vi "Digital Audio Protocol Settings Dialog.vi"() -> (3 "digital audio protocol settings":T1={"number of channels"=0, "data justification"=enum."Left Justified", "endianness"=enum."LSB First", "channel length"=0, "bit depth"=0, "frame clock rate"=0.0, "bit clock edge sync"=enum."Falling", "master clock rate"=0.0, "Logic Level"=enum."1.2 V", "frame sync edge for channel 0"=enum."Rising", "Channel 0 Offset"=0})   [LabVIEW 2021]
uses:
  digital audio protocol settings.ctl
  <vilib>/PDM Acquisition Toolkit/shared/controls/PCM Data Justification.ctl
  <vilib>/PDM Acquisition Toolkit/shared/controls/PCM Bit Endianness.ctl
  <vilib>/PDM Acquisition Toolkit/shared/controls/Digital Edge.ctl
  <vilib>/PDM Acquisition Toolkit/host/Classes/Session/Controls/Logic Levels.ctl
  Program Files/National Instruments/LabVIEW 2021/examples/Digital Audio Acquisition and Generation Toolkit/subVIs/PCM Interface Type.ctl
  <vilib>/PDM Acquisition Toolkit/shared/PDM Shared.lvlib
  <vilib>/PDM Acquisition Toolkit/host/Classes/Session/DecoderSession.lvclass
panel:
  in  "Logic level":enum8{"3.3 V", "1.8 V", "1.2 V"}(ring)=enum."1.8 V"
  in  "Master clock rate":dbl=64.0 format="%#_6pHz"
  out "Bit clock rate":dbl=64.0 format="%#_6pHz"
  in  "Number of channels":u8=2
  in  "TDM":bool
  in  "RJ":bool
  in  "LJ":bool
  in  "I2S":bool
  in  "Bit clock edge  sync":enum8{"Rising", "Falling"}(ring)=enum."Falling"
  in  "Frame clock rate":dbl=64.0 format="%#_6pHz"
  in  "Data Justification":enum16{"Left Justified", "Right Justified"}(ring) caption="Data justification"
  in  "Endianness":enum16{"MSB First", "LSB First"}(ring)
  in  "Bit depth":u8=24
  in  "Channel length":u16=32
  in  "Frame sync edge for Channel 0":enum16{"Rising", "Falling"}(ring)=enum."Falling"
  # "Protocols"
  # "Audio Configuration"
  # "Clock Configuration"
  # "Signal Configuration"
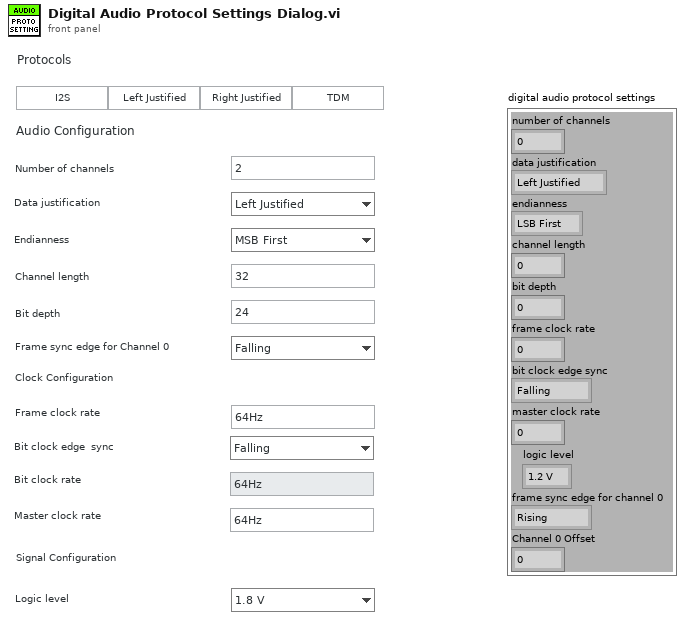
[diagram p1: front panel]
types:
  T1 = typedef "digital audio protocol settings.ctl" = cluster{"number of channels":u16, "data justification":T2, "endianness":T3, "channel length":u16, "bit depth":u8, "frame clock rate":dbl, "bit clock edge sync":T4, "master clock rate":dbl, "Logic Level":T5, "frame sync edge for channel 0":T4, "Channel 0 Offset":u16}
  T2 = typedef "PDM Shared.lvlib/PCM Data Justification.ctl" = enum16{"Left Justified", "Right Justified"}
  T3 = typedef "PDM Shared.lvlib/PCM Bit Endianness.ctl" = enum16{"MSB First", "LSB First"}
  T4 = typedef "PDM Shared.lvlib/Digital Edge.ctl" = enum8{"Rising", "Falling"}
  T5 = typedef "PDM Acquisition Class Library.lvlib/DecoderSession.lvclass/Logic Levels.ctl" = enum16{"3.3 V", "1.8 V", "1.2 V"}
  T6 = enum32{"Invalid", "Standard", "Closed", "Hidden", "Minimized", "Maximized"}
  T7 = typedef "PCM Interface Type.ctl" = enum16{"I2S", "Left Justified", "Right Justified", "TDM 4 Channel", "TDM 6 Channel", "TDM 8 Channel", "DSP mode", "DSP mode with 1 bit delay", "PCM Short Frame", "PCM Long Frame"}
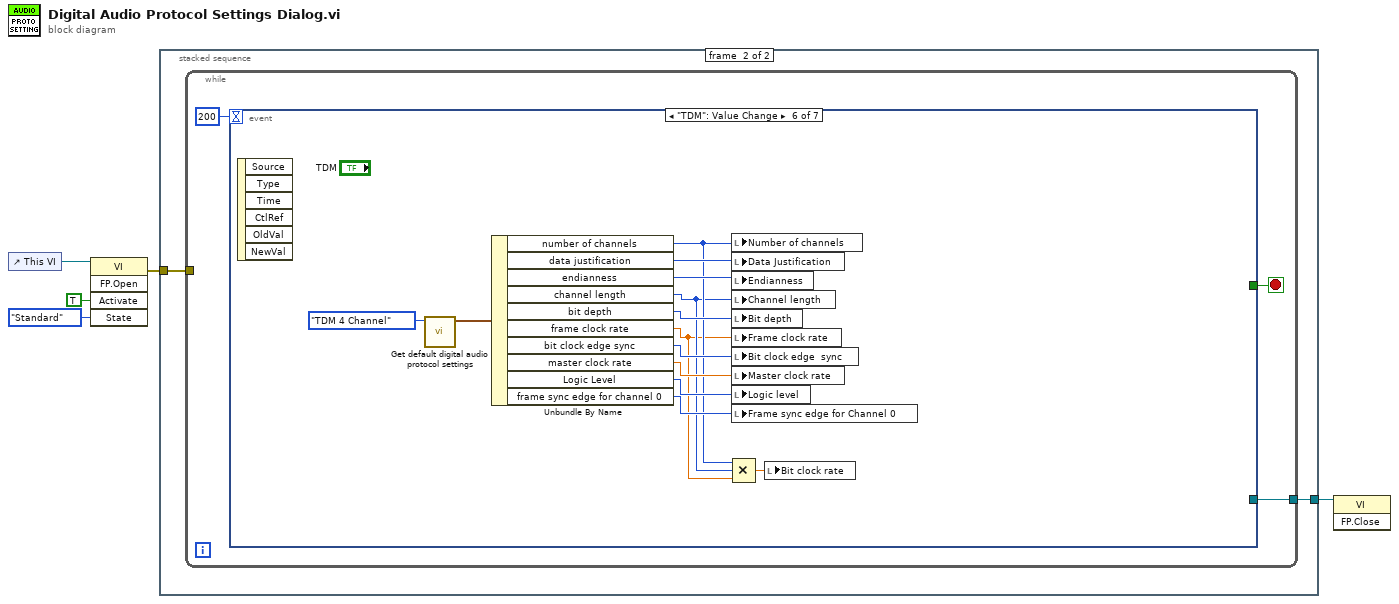
[diagram p0: block diagram]
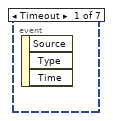
[diagram p3: hidden frame]
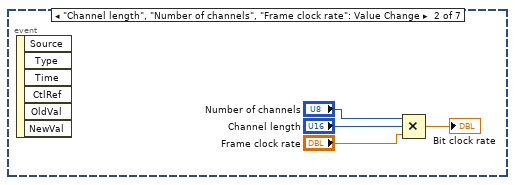
[diagram p4: hidden frame]
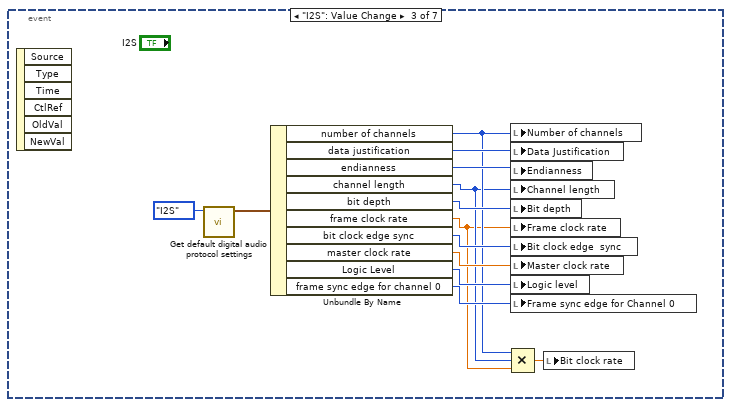
[diagram p5: hidden frame]
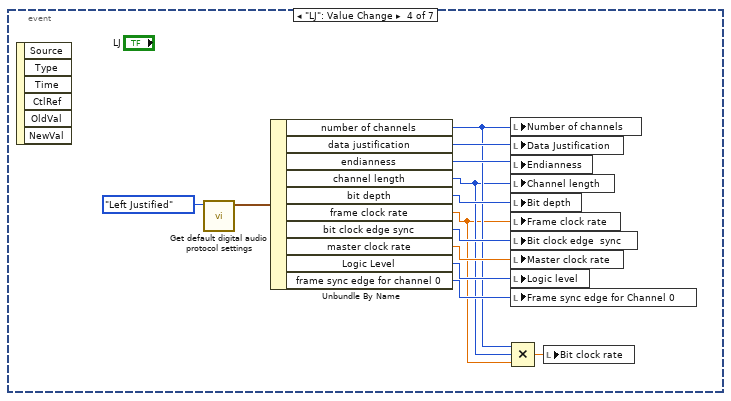
[diagram p6: hidden frame]
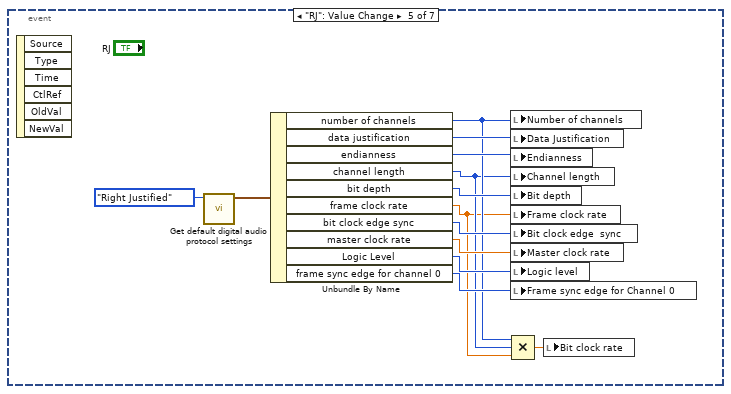
[diagram p7: hidden frame]
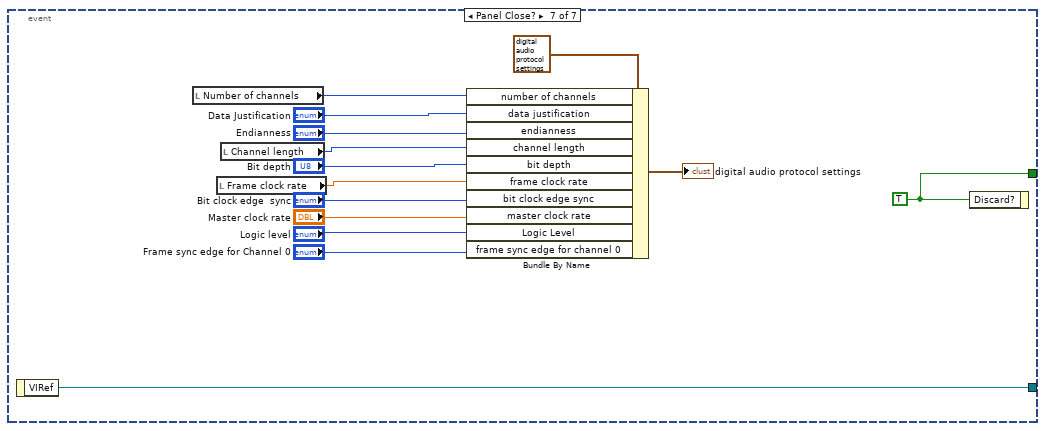
[diagram p8: hidden frame]
diagram:
  n1 = control-ref of="This VI"() -> (w3:refnum<vi>)
  n2 = invoke class="VI" method="FP.Open"(reference=w3, "Activate"=TRUE ("Activate?"), "State"=T6."Standard") -> (error out=w2:errorcluster)  [unwired: 2 in, 4 out]
  n3 = stacked-sequence {
    tunnel: w2 -> [_ w7]
    tunnel: [_ w6] -> w1
    frame #0 {
    }
    frame #1 {
      n4 = while {
        tunnel: [w8] -> w6
        tunnel: w7 -> [_]
        stop <- w10 stop-if-true
        n5 = event shown="[5] \"TDM\": Value Change" {
          selector: _ -> [_ _ _ _ _ _ _]
          dyn-events: _ -> [_ _ _ _ _ _ _]
          timeout: 200 -> [_ _ _ _ _ _ _]
          tunnel: [_ _ _ _ _ _ w79] -> w10
          tunnel: [_ _ _ _ _ _ w80] -> w8
          event Timeout {
            n6 = event-data() -> ()  [unwired: 1 in, 3 out]
          }
          event "Channel length", "Number of channels", "Frame clock rate": Value Change {
            n7 = event-data() -> ()  [unwired: 1 in, 6 out]
            n8 = Compound Arithmetic op=MULTIPLY("Number of channels", "Channel length", "Frame clock rate") -> (→"Bit clock rate":dbl)
          }
          event "I2S": Value Change {
            n9 = event-data() -> ()  [unwired: 1 in, 6 out]
            n10 = call "Get default digital audio protocol settings.vi"("PCM Interfaces"=PCM_Interface_Type."I2S") -> ("digital audio protocol settings"=w27:T1)  [unwired: 10 in]
            n11 = Unbundle By Name(w27) -> ("number of channels"=w18:u16, "data justification"=w25:T2, "endianness"=w24:T3, "channel length"=w17:u16, "bit depth"=w23:u8, "frame clock rate"=w16:dbl, "bit clock edge sync"=w22:T4, "master clock rate"=w21:dbl, "Logic Level"=w20:T5, "frame sync edge for channel 0"=w19:T4)
            n12 = local write "Number of channels"(w18) -> ()
            n13 = local write "Data Justification"(w25) -> ()
            n14 = local write "Endianness"(w24) -> ()
            n15 = local write "Channel length"(w17) -> ()
            n16 = local write "Bit depth"(w23) -> ()
            n17 = local write "Frame clock rate"(w16) -> ()
            n18 = local write "Bit clock edge  sync"(w22) -> ()
            n19 = local write "Master clock rate"(w21) -> ()
            n20 = local write "Logic level"(w20) -> ()
            n21 = local write "Frame sync edge for Channel 0"(w19) -> ()
            n22 = Compound Arithmetic op=MULTIPLY(w18, w17, w16) -> (w15:dbl)
            n23 = local write "Bit clock rate"(w15) -> ()
          }
          event "LJ": Value Change {
            n24 = event-data() -> ()  [unwired: 1 in, 6 out]
            n25 = call "Get default digital audio protocol settings.vi"("PCM Interfaces"=PCM_Interface_Type."Left Justified") -> ("digital audio protocol settings"=w40:T1)  [unwired: 10 in]
            n26 = Unbundle By Name(w40) -> ("number of channels"=w31:u16, "data justification"=w38:T2, "endianness"=w37:T3, "channel length"=w30:u16, "bit depth"=w36:u8, "frame clock rate"=w29:dbl, "bit clock edge sync"=w35:T4, "master clock rate"=w34:dbl, "Logic Level"=w33:T5, "frame sync edge for channel 0"=w32:T4)
            n27 = local write "Number of channels"(w31) -> ()
            n28 = local write "Data Justification"(w38) -> ()
            n29 = local write "Endianness"(w37) -> ()
            n30 = local write "Channel length"(w30) -> ()
            n31 = local write "Bit depth"(w36) -> ()
            n32 = local write "Frame clock rate"(w29) -> ()
            n33 = local write "Bit clock edge  sync"(w35) -> ()
            n34 = local write "Master clock rate"(w34) -> ()
            n35 = local write "Logic level"(w33) -> ()
            n36 = local write "Frame sync edge for Channel 0"(w32) -> ()
            n37 = Compound Arithmetic op=MULTIPLY(w31, w30, w29) -> (w28:dbl)
            n38 = local write "Bit clock rate"(w28) -> ()
          }
          event "RJ": Value Change {
            n39 = event-data() -> ()  [unwired: 1 in, 6 out]
            n40 = call "Get default digital audio protocol settings.vi"("PCM Interfaces"=PCM_Interface_Type."Right Justified") -> ("digital audio protocol settings"=w53:T1)  [unwired: 10 in]
            n41 = Unbundle By Name(w53) -> ("number of channels"=w44:u16, "data justification"=w51:T2, "endianness"=w50:T3, "channel length"=w43:u16, "bit depth"=w49:u8, "frame clock rate"=w42:dbl, "bit clock edge sync"=w48:T4, "master clock rate"=w47:dbl, "Logic Level"=w46:T5, "frame sync edge for channel 0"=w45:T4)
            n42 = local write "Number of channels"(w44) -> ()
            n43 = local write "Data Justification"(w51) -> ()
            n44 = local write "Endianness"(w50) -> ()
            n45 = local write "Channel length"(w43) -> ()
            n46 = local write "Bit depth"(w49) -> ()
            n47 = local write "Frame clock rate"(w42) -> ()
            n48 = local write "Bit clock edge  sync"(w48) -> ()
            n49 = local write "Master clock rate"(w47) -> ()
            n50 = local write "Logic level"(w46) -> ()
            n51 = local write "Frame sync edge for Channel 0"(w45) -> ()
            n52 = Compound Arithmetic op=MULTIPLY(w44, w43, w42) -> (w41:dbl)
            n53 = local write "Bit clock rate"(w41) -> ()
          }
          event "TDM": Value Change {
            n54 = event-data() -> ()  [unwired: 1 in, 6 out]
            n55 = call "Get default digital audio protocol settings.vi"("PCM Interfaces"=PCM_Interface_Type."TDM 4 Channel") -> ("digital audio protocol settings"=w66:T1)  [unwired: 10 in]
            n56 = Unbundle By Name(w66) -> ("number of channels"=w57:u16, "data justification"=w64:T2, "endianness"=w63:T3, "channel length"=w56:u16, "bit depth"=w62:u8, "frame clock rate"=w55:dbl, "bit clock edge sync"=w61:T4, "master clock rate"=w60:dbl, "Logic Level"=w59:T5, "frame sync edge for channel 0"=w58:T4)
            n57 = local write "Number of channels"(w57) -> ()
            n58 = local write "Data Justification"(w64) -> ()
            n59 = local write "Endianness"(w63) -> ()
            n60 = local write "Channel length"(w56) -> ()
            n61 = local write "Bit depth"(w62) -> ()
            n62 = local write "Frame clock rate"(w55) -> ()
            n63 = local write "Bit clock edge  sync"(w61) -> ()
            n64 = local write "Master clock rate"(w60) -> ()
            n65 = local write "Logic level"(w59) -> ()
            n66 = local write "Frame sync edge for Channel 0"(w58) -> ()
            n67 = Compound Arithmetic op=MULTIPLY(w57, w56, w55) -> (w54:dbl)
            n68 = local write "Bit clock rate"(w54) -> ()
          }
          event Panel Close? {
            w79 = TRUE ("Discard?")
            n69 = event-data() -> ("VIRef"=w80:refnum<vi>)  [unwired: 1 in]
            n70 = local read "Number of channels"() -> (w67:u8)
            n71 = local read "Frame clock rate"() -> (w69:dbl)
            n72 = local read "Channel length"() -> (w68:u16)
            n73 = Bundle By Name(cluster=T1 {"number of channels"=0, "data justification"=enum."Left Justified", "endianness"=enum."LSB First", "channel length"=0, "bit depth"=0, "frame clock rate"=0.0, "bit clock edge sync"=enum."Falling", "master clock rate"=0.0, "Logic Level"=enum."1.2 V", "frame sync edge for channel 0"=enum."Rising", "Channel 0 Offset"=0} ("digital audio protocol settings"), "number of channels"=w67, "data justification"="Data Justification", "endianness"="Endianness", "channel length"=w68, "bit depth"="Bit depth", "frame clock rate"=w69, "bit clock edge sync"="Bit clock edge  sync", "master clock rate"="Master clock rate", "Logic Level"="Logic level", "frame sync edge for channel 0"="Frame sync edge for Channel 0") -> (→"digital audio protocol settings":T1)
            n74 = event-data("Discard?"=w79) -> ()  [unwired: 1 in, 1 out]
          }
        }
      }
    }
  }
  n75 = invoke class="VI" method="FP.Close"(reference=w1) -> ()  [unwired: 2 in, 3 out]
